vi "Step Association Add.vi"(8 "error in (no error)":errorcluster, 10 "Step Association Record (empty)":T1, 11 "Connection Refnum":T2) -> (0 "error out":errorcluster, 3 "Connection Refnum":T2)   [LabVIEW 2011]
uses:
  Summitek EXT/ODBC/SQL Controls/Connection Refnum.ctl
  Step Association Record.ctl
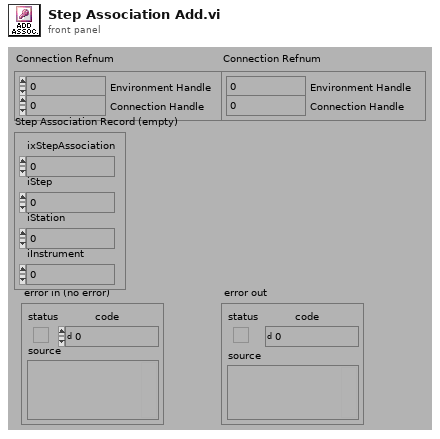
[diagram p1: front panel]
types:
  T1 = typedef "Step Association Record.ctl" = cluster{"ixStepAssociation":i32, "iStep":i32, "iStation":i32, "iInstrument":i32}
  T2 = typedef "Connection Refnum.ctl" = cluster{"Environment Handle":i32, "Connection Handle":i32}
  T3 = typedef "Statement Refnum.ctl" = cluster{"Statement Handle":i32, "Parameter Number":u16}
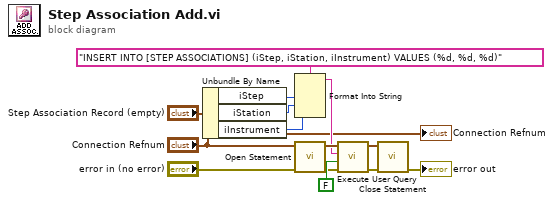
[diagram p0: block diagram]
diagram:
  n1 = Unbundle By Name("Step Association Record (empty)") -> ("iStep"=w3:i32, "iStation"=w2:i32, "iInstrument"=w1:i32)
  n2 = Format Into String(format string="INSERT INTO [STEP ASSOCIATIONS] (iStep, iStation, iInstrument) VALUES (%d, %d, %d)" ("User Query"), w3, w2, w1) -> (resulting string=w8:string)  [unwired: 2 in, 1 out]
  n3 = call "Open Statement.vi"("error in (no error)"="error in (no error)", "Connection Refnum"="Connection Refnum") -> ("error out"=w11:errorcluster, "Statement Refnum"=w10:T3)  [unwired: 4 out]
  n4 = call "Execute User Query.vi"("error in (no error)"=w11, "Return Data? (f)"=FALSE, "User Query"=w8, "Statement Refnum"=w10) -> ("error out"=w12:errorcluster, "Statement Refnum"=w13:T3)  [unwired: 2 out]
  n5 = call "Close Statement.vi"("error in (no error)"=w12, "Statement Refnum"=w13) -> ("error out"=→"error out":errorcluster)  [unwired: 5 out]
  "Connection Refnum" <- "Connection Refnum"
